vi "220506_Basic3.vi"() -> ()   [LabVIEW 2021]
uses:
  <vilib>/numeric/Random Number (Range) DBL.vi
panel:
  out "Temperatur":dbl[](array[numeric])
  out "Numeric":i32
  in  "Values":dbl
  out "Array":dbl[](array[numeric])
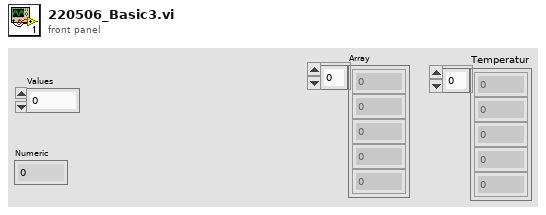
[diagram p1: front panel]
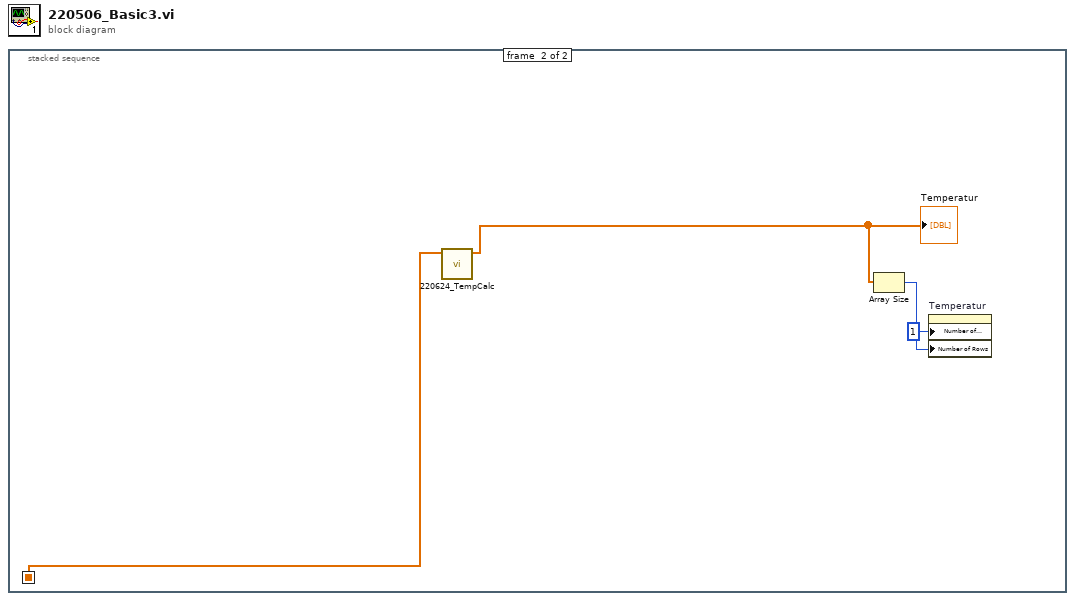
[diagram p0: block diagram]
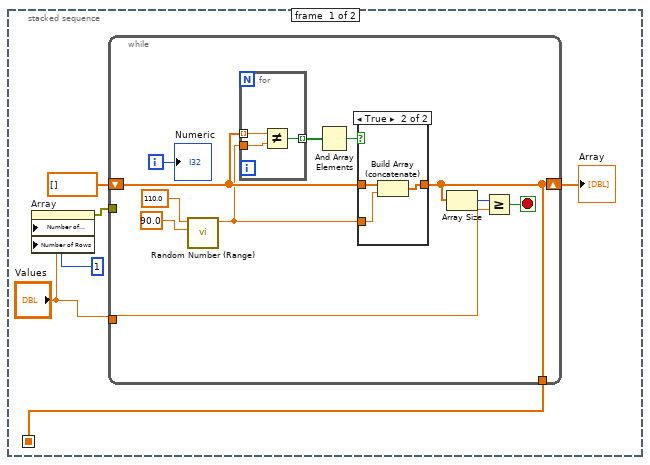
[diagram p2: hidden frame]
diagram:
  n1 = stacked-sequence {
    seq-local: [w1 _] -> [_ w28]
    frame #0 {
      n2 = property on="Array" class="Arr (strict)"("Number of Columns"=u32 1, "Number of Rows"="Values") -> (error out=w2:errorcluster)  [unwired: 2 in, 1 out]
      n3 = while {
        shift-right: [w7] -> w5
        shift-left: dbl[] [] -> [w13]
        tunnel: "Values" -> [w9]
        tunnel: w2 -> [_]
        tunnel: [w7] -> w1
        i -> [w8]
        stop <- w10 stop-if-true
        n4 = call-poly <vilib>:"Random Number (Range).vi"("lower bound (0)"=90.0, "upper bound (100)"=110.0) -> ("number"=w12:dbl)  [unwired: 9 in]
        n5 = for {
          tunnel: w13 -> [w23] mode=indexing
          tunnel: w12 -> [w24]
          tunnel: [w22] -> w15 mode=indexing
          n6 = Not Equal?(x=w23, y=w24) -> (x != y?=w22:bool)
        }
        n7 = And Array Elements(Boolean array=w15) -> (logical AND=w14:bool)
        n8 = case shown="True" w14 {
          tunnel: [w18 w21] -> w7
          tunnel: w13 -> [w18 w20]
          tunnel: w12 -> [_ w19]
          frame False {
          }
          frame True {
            n9 = Build Array (concatenate)(w20, w19) -> (w21:dbl[])
          }
        }
        n10 = Array Size(array=w7) -> (size(s)=w11:i32)
        n11 = Greater Or Equal?(x=w11, y=w9) -> (x >= y?=w10:bool)
        "Numeric" <- w8
      }
      "Array" <- w5
    }
    frame #1 {
      n12 = call "220624_TempCalc.vi"("R-Values"=w28) -> ("Temp"=w27:dbl[])  [unwired: 10 in]
      "Temperatur" <- w27
      n13 = Array Size(array=w27) -> (size(s)=w26:i32)
      n14 = property on="Temperatur" class="Arr (strict)"("Number of Columns"=u32 1, "Number of Rows"=w26) -> ()  [unwired: 2 in, 2 out]
    }
  }
